vi "_Sample Generator+Set freq+optimal.vi"() -> ()   [LabVIEW 2014]
panel:
  out "elemszam":dbl
  in  "periods":u8=1
  out "tmr 2 rld value":u16
  in  "Signal freq [Hz]":u32
  out "VISA Refnum out":refnum<visa-resource-name>
  out "error out":errorcluster
  in  "VISA resource name":refnum<visa-resource-name>
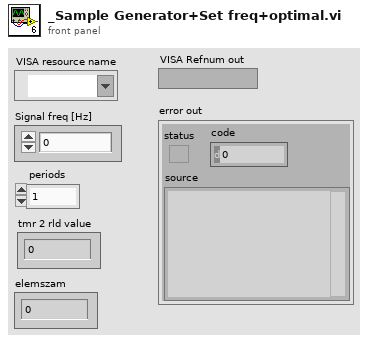
[diagram p1: front panel]
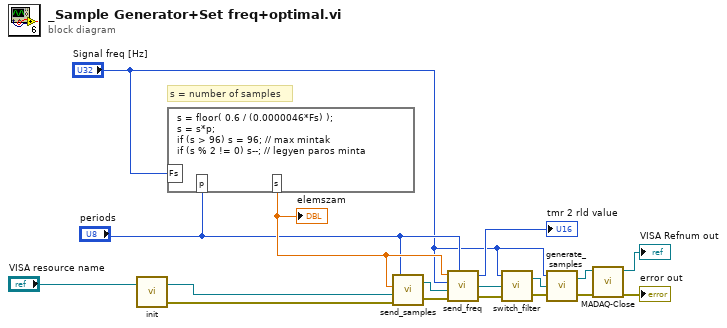
[diagram p0: block diagram]
diagram:
  # "s = number of samples"
  n1 = call "init.vi"("VISA Refnum in"="VISA resource name") -> ("error out"=w6:errorcluster, "VISA Refnum out"=w7:refnum<visa-resource-name>)  [unwired: 1 in]
  n2 = formula code="s = floor( 0.6 / (0.0000046*Fs) );\ns = s*p;\nif (s > 96) s = 96; // max mintak\nif (s % 2 != 0) s--; // legyen paros minta"("Fs"="Signal freq [Hz]", "p"="periods") -> ("s"=w9:dbl)
  "elemszam" <- w9
  n3 = call "send_samples.vi"("error in (no error)"=w6, "VISA Refnum in"=w7, "elemszam"=w9, "periods"="periods") -> ("error out"=w12:errorcluster, "VISA Refnum out"=w10:refnum<visa-resource-name>)
  n4 = call "send_freq.vi"("elemszam"=w9, "signal freq"="Signal freq [Hz]", "VISA Refnum in"=w10, "error in (no error)"=w12, "periods"="periods") -> ("tmr 2 rld value"=→"tmr 2 rld value":u16, "VISA Refnum out"=w5:refnum<visa-resource-name>, "error out"=w4:errorcluster)
  n5 = call "switch_filter.vi"("error in (no error)"=w4, "VISA Refnum in"=w5, "fs"="Signal freq [Hz]") -> ("error out"=w3:errorcluster, "VISA Refnum out"=w2:refnum<visa-resource-name>)
  n6 = call "generate_samples.vi"("error in (no error) 2"=w3, "VISA Refnum in 2"=w2, "fs"="Signal freq [Hz]") -> ("error out"=w13:errorcluster, "VISA Refnum out"=w14:refnum<visa-resource-name>)
  n7 = call "MADAQ-Close.vi"("error in (no error)"=w13, "VISA resource name"=w14) -> ("error out"=→"error out":errorcluster, "VISA resource name out"=→"VISA Refnum out":refnum<visa-resource-name>)  [unwired: 4 in]
